vi "niScope Abort Digitizing on Virtual Channels.vi"(8 "error in":errorcluster, 10 "abort (True)":bool=TRUE, 11 "niScope in":T1={"channel cfg"=[], "sessions"=[], "multi cards"=FALSE, "channels"=0, "type"=enum."n/a", "memory [B/chn]"=0, "ext. clock [Hz]"=0.0, "samples count"=0, "use streaming"=FALSE, "proc setup"={"packet size [smpl]"=0, "current timeout [s]"=0.0, "blk2blk timeout [s]"=0.0, "event time"=timestamp(0 s since 1904-01-01), "temp sampl T [s]"=0.0, "data queue"=refnum, "stop notifier"=refnum, "proc ref"=refnum}, "sample width [B]"=0, "ranges [V]"=[], "trigger setup"={"coupling"=1, "level [V]"=0.0, "slope"=0, "mode"=enum."Immediate"}, "fs [Hz]"=0.0, "bitres [bit]"=0} {"trigger setup"."level [V]" format="%.2f"; "trigger setup"."coupling" items=["AC"=0, "DC"=1, "HF Reject"=3, "LF Reject"=4, "AC Plus HF Reject"=1001]; "channel cfg"."Range [Vpk]" min=0.0; "channel cfg"."Channel" min=0}) -> (0 "error out":errorcluster, 3 "niScope out":T1={"channel cfg"=[], "sessions"=[], "multi cards"=FALSE, "channels"=0, "type"=enum."n/a", "memory [B/chn]"=0, "ext. clock [Hz]"=0.0, "samples count"=0, "use streaming"=FALSE, "proc setup"={"packet size [smpl]"=0, "current timeout [s]"=0.0, "blk2blk timeout [s]"=0.0, "event time"=timestamp(0 s since 1904-01-01), "temp sampl T [s]"=0.0, "data queue"=refnum, "stop notifier"=refnum, "proc ref"=refnum}, "sample width [B]"=0, "ranges [V]"=[], "trigger setup"={"coupling"=1, "level [V]"=0.0, "slope"=0, "mode"=enum."Immediate"}, "fs [Hz]"=0.0, "bitres [bit]"=0} {"trigger setup"."level [V]" format="%.2f"; "trigger setup"."coupling" items=["AC"=0, "DC"=1, "HF Reject"=3, "LF Reject"=4, "AC Plus HF Reject"=1001]; "channel cfg"."Range [Vpk]" min=0.0; "channel cfg"."Channel" min=0})   [LabVIEW 2013, in "niScope Virtual Digitizer.lvlib"]
doc: "Tries to abort digitizing at all virtual channels. The VI ignores input errors and will not generate any additional errors even if the digtizer is no longer running or the instrument references are invalid."
uses:
  niScope Virtual Digitizer.lvlib
  niScope Session.ctl
  niScope Virtual Channel Config.ctl
  niScope Virtual Channel Mode.ctl
  niScope Virtual Channel Input Z.ctl
  niScope Virtual Channel Coupling.ctl
  niScope Type.ctl
  niScope Digitizing Process Options.ctl
  niScope Data Packet.ctl
  niScope Trigger Setup.ctl
  <instrlib>/niScope/Controls/niScope trigger coupling.ctl
  <instrlib>/niScope/Controls/niScope trigger slope.ctl
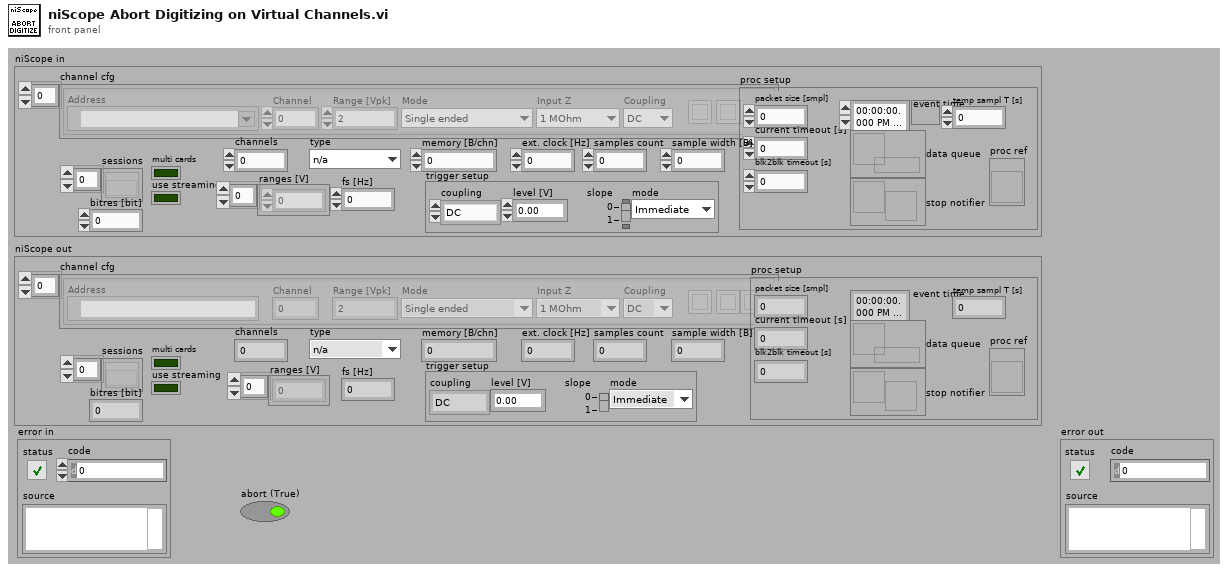
[diagram p1: front panel]
types:
  T1 = typedef "niScope Virtual Digitizer.lvlib/niScope Session.ctl" = cluster{"channel cfg":T2[], "sessions":refnum<k20>[], "multi cards":bool, "channels":i32, "type":T6, "memory [B/chn]":i32, "ext. clock [Hz]":dbl, "samples count":i64, "use streaming":bool, "proc setup":T7, "sample width [B]":i32, "ranges [V]":dbl[], "trigger setup":T8, "fs [Hz]":dbl, "bitres [bit]":i32}
  T2 = typedef "niScope Virtual Digitizer.lvlib/niScope Virtual Channel Config.ctl" = cluster{"Address":refnum<k15>, "Channel":i32, "Mode":T3, "Input Z":T4, "Coupling":T5, "Range [Vpk]":dbl, "btn clr":bool, "btn up":bool, "btn down":bool}
  T3 = typedef "niScope Virtual Digitizer.lvlib/niScope Virtual Channel Mode.ctl" = enum16{"Single ended", "Unbal. differential", "Differential"}
  T4 = typedef "niScope Virtual Digitizer.lvlib/niScope Virtual Channel Input Z.ctl" = enum16{"1 MOhm", "50 Ohm"}
  T5 = typedef "niScope Virtual Digitizer.lvlib/niScope Virtual Channel Coupling.ctl" = enum16{"AC", "DC", "GND"}
  T6 = typedef "niScope Virtual Digitizer.lvlib/niScope Type.ctl" = enum16{"n/a", "5922"}
  T7 = typedef "niScope Virtual Digitizer.lvlib/niScope Digitizing Process Options.ctl" = cluster{"packet size [smpl]":i64, "current timeout [s]":dbl, "blk2blk timeout [s]":dbl, "event time":timestamp, "temp sampl T [s]":dbl, "data queue":refnum<queue>, "stop notifier":refnum<notifier>, "proc ref":refnum<vi>}
  T8 = typedef "niScope Virtual Digitizer.lvlib/niScope Trigger Setup.ctl" = cluster{"coupling":T9, "level [V]":dbl, "slope":T10, "mode":enum16{"Immediate", "External", "Level"}}
  T9 = typedef "niScope trigger coupling.ctl" = u16
  T10 = typedef "niScope trigger slope.ctl" = i32
  T11 = typedef "niScope Virtual Digitizer.lvlib/niScope Physical Cards.ctl" = cluster{"chn lst":i32[], "addr":refnum<k15>, "chn pos":i32[]}
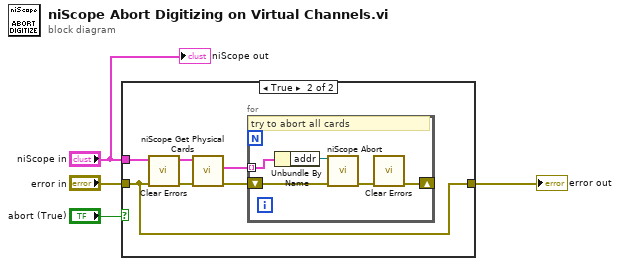
[diagram p0: block diagram]
diagram:
  n1 = case shown="True" "abort (True)" {
    tunnel: "error in" -> [w5 w6]
    tunnel: "niScope in" -> [_ w8]
    tunnel: [w5 w6] -> w4
    frame False {
    }
    frame True {
      n2 = call <vilib>:"Clear Errors.vi"("error in (no error)"=w6) -> ("error out"=w7:errorcluster)  [unwired: 6 in]
      n3 = call "niScope Get Physical Cards.vi"("error in"=w7, "niScope in"=w8) -> ("error out"=w10:errorcluster, "card list"=w9:T11[])  [unwired: 7 in, 1 out]
      n4 = for {
        tunnel: w9 -> [w15] mode=indexing
        shift-right: [w11] -> _
        shift-left: w10 -> [w13]
        # "try to abort all cards"
        n5 = Unbundle By Name(w15) -> ("addr"=w14:refnum<k15>)
        n6 = call <instrlib>:"niScope Abort.vi"("instrument handle"=w14, "error in"=w13) -> ("error out"=w12:errorcluster)  [unwired: 12 in, 1 out]
        n7 = call <vilib>:"Clear Errors.vi"("error in (no error)"=w12) -> ("error out"=w11:errorcluster)  [unwired: 6 in]
      }
    }
  }
  "error out" <- w4
  "niScope out" <- "niScope in"
